vi "TcA07-002_SupportMethods.vi"(1 "Input buffer":T3="1", 3 "Invocation info":T2, 5 "error in (no error)":errorcluster, 6 "Add log to result?":bool) -> (16 "Test Data":T1 {"Numeric Measurement" format="%.2f"}, 19 "error out":errorcluster)   [LabVIEW 2020]
doc: "Test case template."
uses:
  Shared/Support_InputBuffer.ctl
  Shared/Support_InvocationInfo.ctl
  Shared/Support_TestData.ctl
  TestClasses/G#BaseClass1_class/G#BaseClass1.lvclass
  TestClasses/G#SubSubClass1_class/G#SubSubClass1.lvclass
  TestClasses/G#BaseClass2_class/G#BaseClass2.lvclass
  <vilib>/addons/_AddQ/G#Object/G#Object.lvclass
  TestClasses/G#SubClass2_class/G#SubClass2.lvclass
  TestClasses/G#SubClass1_class/G#SubClass1.lvclass
panel:
  in  "Test name":string="TcA07-002 Support Methods"
  out "Test result":bool
  out "Result":string
  # "Verify that the support methods works as expected."
  # "Sub test case"
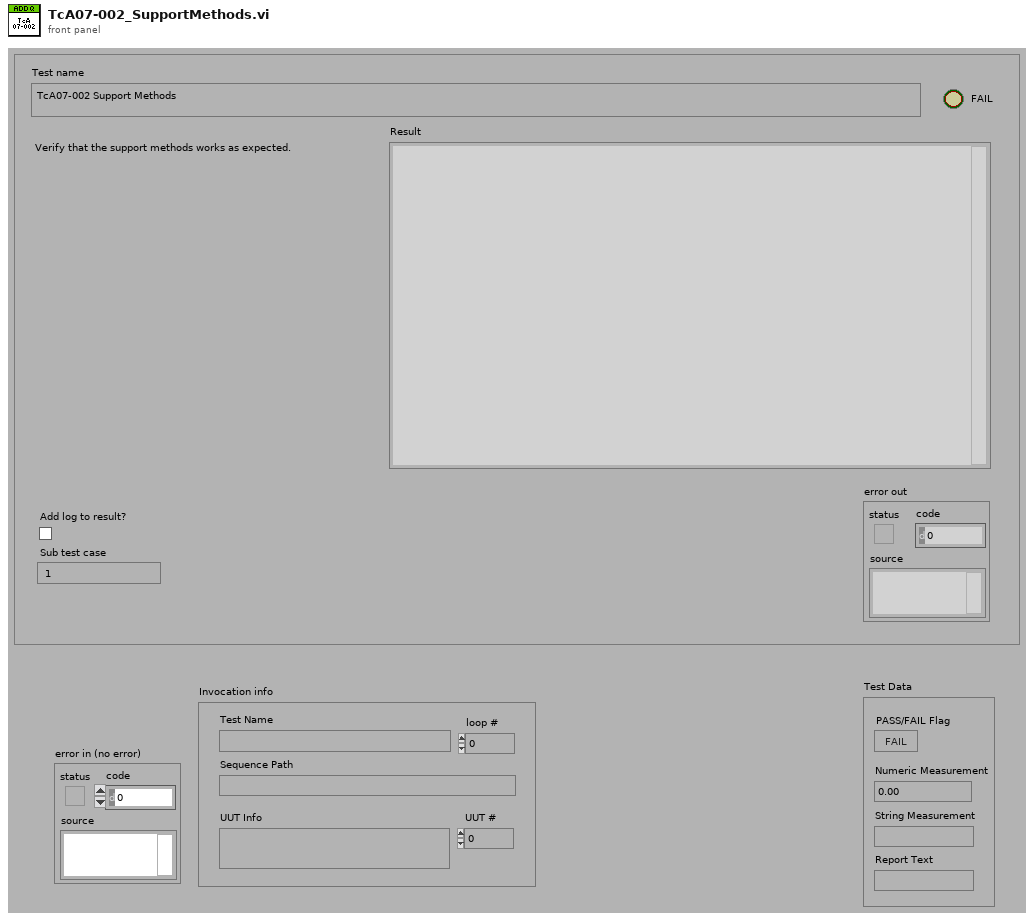
[diagram p1: front panel]
types:
  T1 = typedef "Support_TestData.ctl" = cluster{"PASS/FAIL Flag":bool, "Numeric Measurement":dbl, "String Measurement":string, "Report Text":string}
  T2 = typedef "Support_InvocationInfo.ctl" = cluster{"UUT #":i32, "loop #":i32, "UUT Info":string, "Test Name":string, "Sequence Path":path}
  T3 = typedef "Support_InputBuffer.ctl" = string
  T4 = typedef "Support_ResultType.ctl" = cluster{"Pass":bool, "Comment":string, "MeasurementValue":dbl}
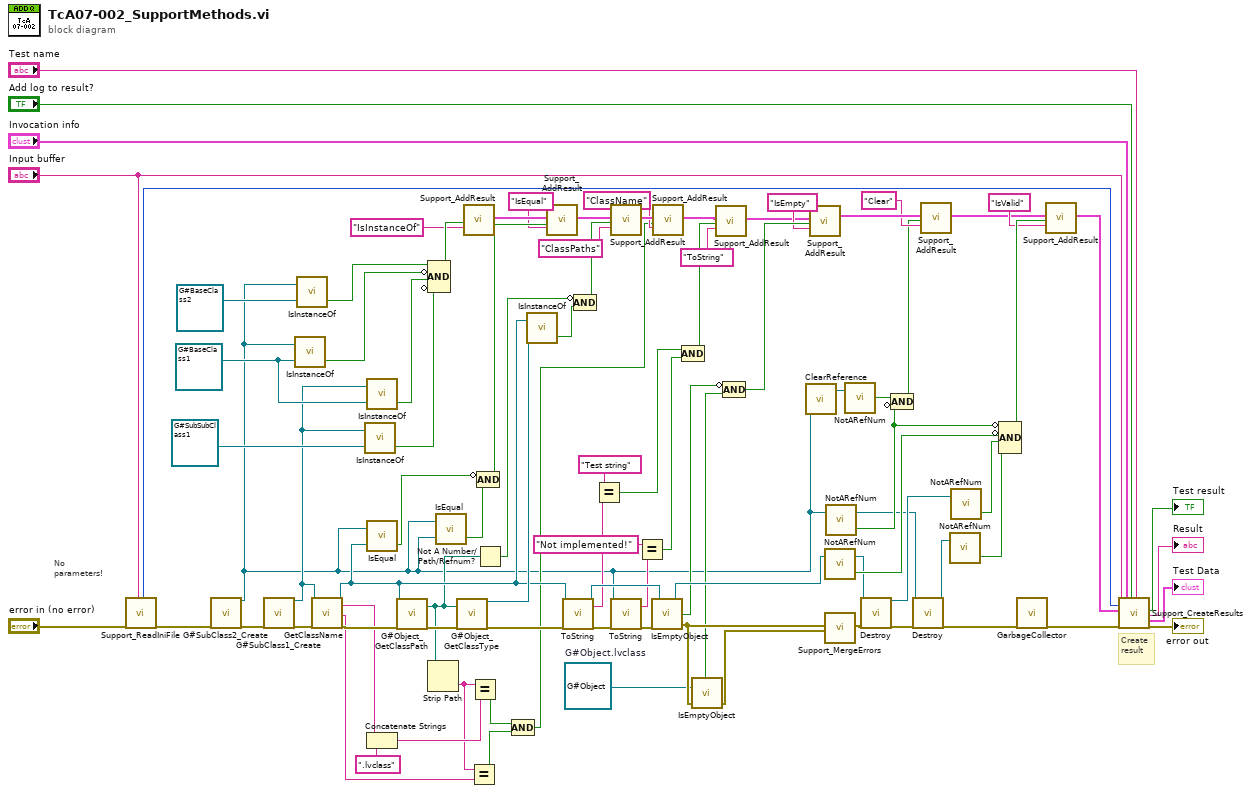
[diagram p0: block diagram]
diagram:
  w4 = refnum<class "G#Object.lvclass"> refnum  # G#Object.lvclass
  w75 = refnum<class "G#BaseClass1.lvclass"> refnum ("G#BaseClass1.lvclass")
  # "No\nparameters!"
  # "Create\nresult"
  n1 = call "Support_ReadIniFile.vi"("error in (no error)"="error in (no error)", "Sub test case"="Input buffer") -> ("Timer start"=w83:u32, "error out"=w81:errorcluster)  [unwired: 10 in, 6 out]
  n2 = call "G#SubClass2_Create.vi"("error in (no error)"=w81) -> ("reference out"=w3:refnum<class "G#SubClass2.lvclass">, "error out"=w80:errorcluster)  [unwired: 17 in]
  n3 = call "G#SubClass1_Create.vi"("error in (no error)"=w80) -> ("reference out"=w73:refnum<class "G#SubClass1.lvclass">, "error out"=w77:errorcluster)  [unwired: 16 in, 1 out]
  n4 = call-dynamic "IsInstanceOf.vi"("is object instance of"=w75, "reference in"=w3) -> ("is instance of"=w71:bool)  [unwired: 1 out]
  n5 = call-dynamic "IsInstanceOf.vi"("is object instance of"=refnum<class "G#BaseClass2.lvclass"> refnum ("G#BaseClass2.lvclass"), "reference in"=w3) -> ("is instance of"=w72:bool)  [unwired: 1 out]
  n6 = call-dynamic "GetClassName.vi"("reference in"=w73, "error in (no error)"=w77) -> ("reference out"=w40:refnum<class "G#SubClass1.lvclass">, "class name"=w33:string, "full class name"=w29:string, "error out"=w44:errorcluster)  [unwired: 13 in, 1 out]
  n7 = call-dynamic "IsInstanceOf.vi"("is object instance of"=refnum<class "G#SubSubClass1.lvclass"> refnum ("G#SubSubClass1.lvclass"), "reference in"=w73) -> ("is instance of"=w69:bool)  [unwired: 1 out]
  n8 = call-dynamic "IsInstanceOf.vi"("is object instance of"=w75, "reference in"=w73) -> ("is instance of"=w70:bool)  [unwired: 1 out]
  n9 = call-dynamic "IsEqual.vi"("is equal to"=w40, "reference in"=w3) -> ("is equal"=w49:bool)  [unwired: 1 out]
  n10 = Concatenate Strings(w33, ".lvclass" ("string")) -> (w31:string)
  n11 = call-dynamic "G#Object_GetClassPath.vi"("reference in"=w40, "error in (no error)"=w44) -> ("class path"=w34:path, "error out"=w43:errorcluster)  [unwired: 15 in, 1 out]
  n12 = Compound Arithmetic op=AND(w72, invert w71, w70, invert w69) -> (w68:bool)
  n13 = Strip Path(path=w34) -> (name=w30:string)  [unwired: 1 out]
  n14 = call-dynamic "IsEqual.vi"("is equal to"=w3, "reference in"=w3) -> ("is equal"=w48:bool)  [unwired: 1 out]
  n15 = call <vilib>:"G#Object_GetClassType.vi"("class path"=w34, "error in (no error)"=w43) -> ("reference out"=w42:refnum<class "G#Object.lvclass">, "error out"=w41:errorcluster)  [unwired: 16 in]
  n16 = call "Support_AddResult.vi"("Pass"=w68, "Comment"="IsInstanceOf") -> ("Results out"=w47:T4[])  [unwired: 17 in]
  n17 = Equal?(x=w30, y=w29) -> (x = y?=w27:bool)
  n18 = Equal?(x=w30, y=w31) -> (x = y?=w28:bool)
  n19 = Not A Number/Path/Refnum?(number/path/refnum=w34) -> (NaN/Path/Refnum?=w36:bool)
  n20 = Compound Arithmetic op=AND(invert w49, w48) -> (w46:bool)
  n21 = Compound Arithmetic op=AND(w28, w27) -> (w5:bool)
  n22 = call-dynamic "IsInstanceOf.vi"("is object instance of"=w42, "reference in"=w40) -> ("is instance of"=w37:bool)  [unwired: 1 out]
  n23 = call "Support_AddResult.vi"("Results in"=w47, "Pass"=w46, "Comment"="IsEqual") -> ("Results out"=w38:T4[])  [unwired: 16 in]
  n24 = call-dynamic "ToString.vi"("reference in"=w40, "error in (no error)"=w41) -> ("reference out"=w39:refnum<class "G#SubClass1.lvclass">, "string"=w24:string, "error out"=w23:errorcluster)  [unwired: 15 in]
  n25 = Compound Arithmetic op=AND(invert w36, w37) -> (w7:bool)
  n26 = Equal?(x="Test string", y=w24) -> (x = y?=w19:bool)
  n27 = call "Support_AddResult.vi"("Results in"=w38, "Pass"=w7, "Comment"="ClassPaths") -> ("Results out"=w8:T4[])  [unwired: 16 in]
  n28 = call-dynamic "ToString.vi"("reference in"=w3, "error in (no error)"=w23) -> ("string"=w21:string, "error out"=w22:errorcluster)  [unwired: 15 in, 1 out]
  n29 = Equal?(x="Not implemented!", y=w21) -> (x = y?=w18:bool)
  n30 = call-dynamic "IsEmptyObject.vi"("error in (no error)"=w22, "reference in"=w39) -> ("error out"=w58:errorcluster, "is empty?"=w56:bool, "reference out"=w61:refnum<class "G#SubClass1.lvclass">)  [unwired: 1 in]
  n31 = call "Support_AddResult.vi"("Results in"=w8, "Pass"=w5, "Comment"="ClassName") -> ("Results out"=w9:T4[])  [unwired: 16 in]
  n32 = Compound Arithmetic op=AND(w19, w18) -> (w17:bool)
  n33 = call-dynamic "IsEmptyObject.vi"("error in (no error)"=w58, "reference in"=w4) -> ("error out"=w57:errorcluster, "is empty?"=w55:bool)  [unwired: 1 in, 1 out]
  n34 = call "Support_AddResult.vi"("Results in"=w9, "Pass"=w17, "Comment"="ToString") -> ("Results out"=w26:T4[])  [unwired: 16 in]
  n35 = Compound Arithmetic op=AND(invert w56, w55) -> (w54:bool)
  n36 = call-dynamic "ClearReference.vi"("reference in"=w3) -> ("reference out"=w59:refnum<class "G#SubClass2.lvclass">)
  n37 = call "Support_AddResult.vi"("Results in"=w26, "Pass"=w54, "Comment"="IsEmpty") -> ("Results out"=w15:T4[])  [unwired: 16 in]
  n38 = call-dynamic "NotARefNum.vi"("reference in"=w61) -> ("not a refnum?"=w64:bool, "reference out"=w2:refnum<class "G#SubClass1.lvclass">)  [unwired: 1 in]
  n39 = call "Support_MergeErrors.vi"("error in 1"=w58, "error in 2"=w57) -> ("error out"=w60:errorcluster)  [unwired: 16 in, 1 out]
  n40 = call-dynamic "NotARefNum.vi"("reference in"=w3) -> ("not a refnum?"=w12:bool, "reference out"=w1:refnum<class "G#SubClass2.lvclass">)  [unwired: 1 in]
  n41 = call-dynamic "NotARefNum.vi"("reference in"=w59) -> ("not a refnum?"=w11:bool)  [unwired: 1 in, 1 out]
  n42 = call-dynamic "Destroy.vi"("reference in"=w2, "error in (no error)"=w60) -> ("reference out"=w66:refnum<class "G#SubClass1.lvclass">, "error out"=w78:errorcluster)  [unwired: 16 in]
  n43 = Compound Arithmetic op=AND(w11, invert w12) -> (w10:bool)
  n44 = call-dynamic "Destroy.vi"("reference in"=w1, "error in (no error)"=w78) -> ("reference out"=w65:refnum<class "G#SubClass2.lvclass">, "error out"=w79:errorcluster)  [unwired: 16 in]
  n45 = call "Support_AddResult.vi"("Results in"=w15, "Pass"=w10, "Comment"="Clear") -> ("Results out"=w14:T4[])  [unwired: 16 in]
  n46 = call-dynamic "NotARefNum.vi"("reference in"=w65) -> ("not a refnum?"=w62:bool)  [unwired: 1 in, 1 out]
  n47 = call-dynamic "NotARefNum.vi"("reference in"=w66) -> ("not a refnum?"=w63:bool)  [unwired: 1 in, 1 out]
  n48 = Compound Arithmetic op=AND(invert w12, invert w64, w63, w62) -> (w53:bool)
  n49 = call <vilib>:"GarbageCollector.vi"("error in (no error)"=w79) -> ("error out"=w82:errorcluster)  [unwired: 16 in, 2 out]
  n50 = call "Support_AddResult.vi"("Results in"=w14, "Pass"=w53, "Comment"="IsValid") -> ("Results out"=w52:T4[])  [unwired: 16 in]
  n51 = call "Support_CreateResults.vi"("Sub test case"="Input buffer", "Timer start"=w83, "Results"=w52, "error in (no error)"=w82, "Invocation info"="Invocation info", "Add log to result?"="Add log to result?", "Test name"="Test name") -> ("Pass/fail flag"=→"Test result":bool, "Result"=→"Result":string, "Test Data"=→"Test Data":T1, "error out"=→"error out":errorcluster)  [unwired: 9 in]
